vi "ini_save_variant.vi"(7 "section":string, 8 "error in":errorcluster, 9 "Variant":variant, 10 "key":string, 11 "refnum in":T1) -> (0 "error out":errorcluster, 2 "found?":bool, 3 "refnum out":T1)   [LabVIEW 2018]
uses:
  <vilib>/Utility/config.llb/Config Data RefNum.ctl
  <vilib>/Utility/config.llb/Write Key (String).vi
  <vilib>/Utility/config.llb/NI_LVConfig.lvlib
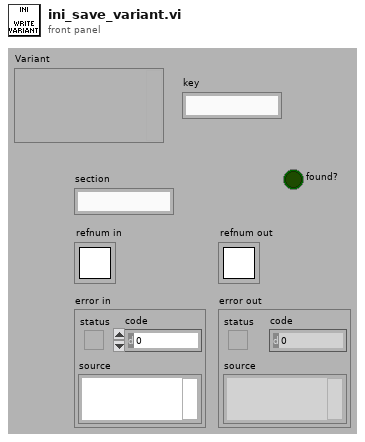
[diagram p1: front panel]
types:
  T1 = typedef "NI_LVConfig.lvlib/Config Data RefNum.ctl" = refnum<k1>
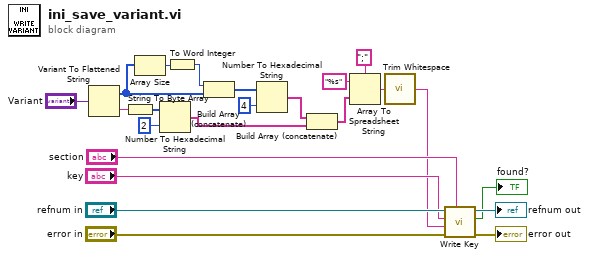
[diagram p0: block diagram]
diagram:
  n1 = Variant To Flattened String(Variant="Variant") -> (data string=w6:string, 1:w13:i16[])
  n2 = String To Byte Array(string=w6) -> (unsigned byte array=w5:u8[])
  n3 = Array Size(array=w13) -> (size(s)=w14:i32)
  n4 = Number To Hexadecimal String(1:i16 2 ("width (-)"), 2:w5) -> (0:w3:string[])
  n5 = To Word Integer(number=w14) -> (16bit integer=w12:i16)
  n6 = Build Array (concatenate)(w12, w13) -> (w11:i16[])
  n7 = Number To Hexadecimal String(1:i16 4 ("width (-)"), 2:w11) -> (0:w8:string[])
  n8 = Build Array (concatenate)(w8, w3) -> (w7:string[])
  n9 = Array To Spreadsheet String(delimiter (Tab)=";", array=w7, 3:"%s" ("format string")) -> (spreadsheet string=w2:string)
  n10 = call <vilib>:"Trim Whitespace.vi"("string"=w2) -> ("trimmed string"=w1:string)  [unwired: 1 in]
  n11 = call-poly <vilib>:"Write Key.vi"("section"="section", "error in (no error)"="error in", "value"=w1, "key"="key", "refnum"="refnum in") -> ("error out"=→"error out":errorcluster, "found?"=→"found?":bool, "refnum out"=→"refnum out":T1)  [unwired: 4 in]
